vi "GUI_HPD_TelescopeStage.vi"() -> ()   [LabVIEW 2011]
uses:
  GUI_Template/GUI_master/tcp_new_data_event.ctl
  GUI_Template/GUI_master/tcp new data cluster.ctl
panel:
  in  "highspeed::1":dbl=0.001 caption="Speed" min=1000.0 max=6000000.0 format="%_4p"
  in  "stop":bool
  in  "position::1":dbl=0.001 caption="Position" min=-5.0 max=25.0 step=1.0 format="%_4p"
  in  "GUIdevice 1":string="HPDTelescopeStage"
  out "tcp data event":T1
  out "error IO 2":errorcluster
  # "HPD Telescope Stage"
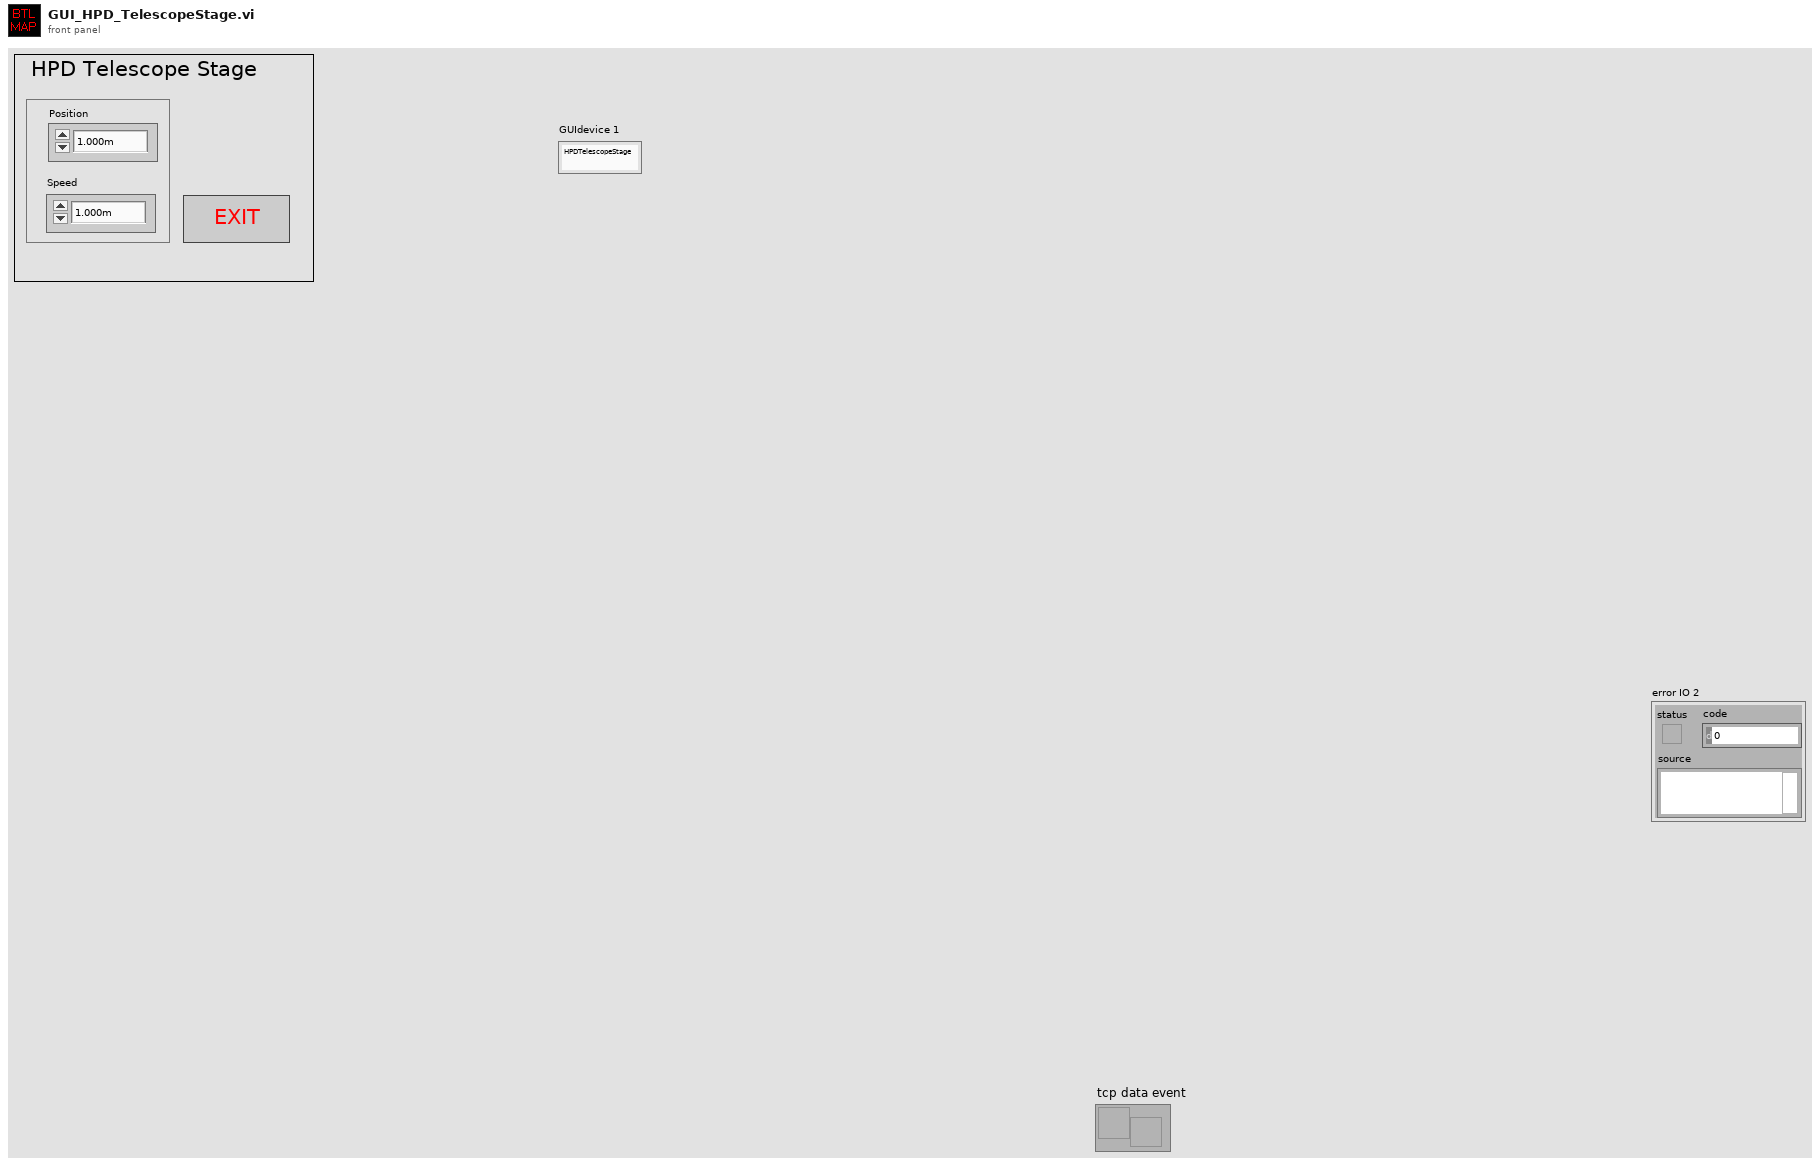
[diagram p1: front panel]
types:
  T1 = typedef "tcp_new_data_event.ctl" = refnum<user-event>
  T2 = typedef "tcp new data cluster.ctl" = cluster{"EventEnum":enum16{"new data", "connection status update"}, "Device name":string}
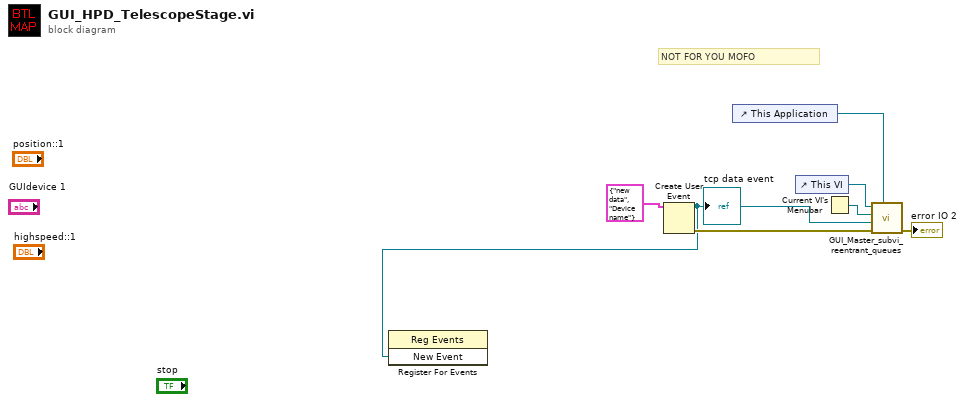
[diagram p0: block diagram]
diagram:
  # "NOT FOR YOU MOFO"
  n1 = Create User Event(user event datatype=T2 {"EventEnum"=enum."new data", "Device name"="Device name"} ("New Event")) -> (user event=w3:refnum<user-event>, error out=w4:errorcluster)  [unwired: 1 in]
  "tcp data event" <- w3
  n2 = register-events(w3) -> ()  [unwired: 2 in, 2 out]
  n3 = control-ref of="This Application"() -> (w1:refnum<vi>)
  n4 = control-ref of="This VI"() -> (w2:refnum<vi>)
  n5 = Current VI's Menubar() -> (w6:refnum<k9>)
  n6 = call "GUI_Master_subvi_reentrant_queues.vi"("This Application"=w1, "error in (no error)"=w4, "tcp data event"=w3, "Caller menu reference"=w6, "Caller VI ref"=w2) -> ("error out"=→"error IO 2":errorcluster)  [unwired: 6 in]
